vi "Backup get fpga resource ref from channels.vi"(0 "bitfile ref in":refnum<k20>, 5 "channel":refnum<class "TBM channel.lvclass">, 11 "error in (no error)":errorcluster) -> (4 "control ref out":refnum<k20>, 6 "fpga res type":T1, 15 "error out":errorcluster)   [LabVIEW 2015]
uses:
  <vilib>/NI/Tag Bus Module Framework/channel/TBM channel.lvclass
  configuration/fpga resource supported data types.ctl
  fpga channel/fpga channel.lvclass
  <vilib>/NI/Tag Bus/tag/tag descriptor.lvclass/tag descriptor.ctl
  fpga channel/fpga channel.lvclass/fpga channel.ctl
  FXP I_20_5.ctl
  FXP I_24_5.ctl
  FXP I_24_10.ctl
  <vilib>/NI/LVFPGA Adv Session Resources/OpenByNameSubVI.vi
  <vilib>/NI/Tag Bus/tag/read tag name.vi
  fpga channel/Read FXP type.vi
  <vilib>/NI/Tag Bus/tag/read data type.vi
  <vilib>/rvi/interface/common/dynamic/niFpgaEscapeDelimiterAndNull.vi
  <vilib>/Utility/error.llb/Error Cluster From Error Code.vi
  <vilib>/NI/LVFPGA Adv Session Resources/OpenByName.xnode
  <vilib>/NI/LVFPGA Adv Session Resources/LVFPGAAdvSessionResources.lvlib
  configuration/io configuration.lvclass
  io runtime.lvclass
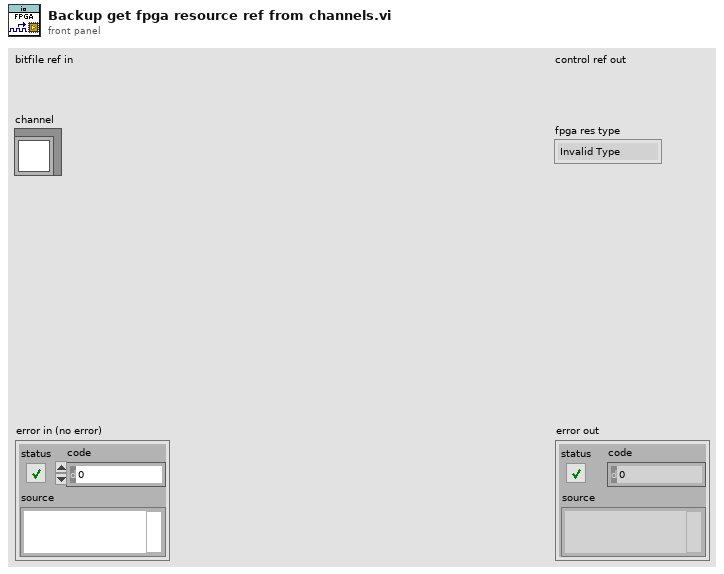
[diagram p1: front panel]
types:
  T1 = typedef "io configuration.lvclass/fpga resource supported data types.ctl" = enum16{"Invalid Type", "Single", "I64", "I32", "I16", "I8", "U64", "U32", "U16", "U8", "Boolean", "FXP I,20,5", "FXP I,24,5", "FXP I,24,10", "Array of I16"}
  T2 = cluster{"Name":string, "Depth":u32, "Write? (Deprecated:Use Implementation)":bool, "Physical Channel":u32, "Base Address":u32, "Data Width":u32, "Data Type":enum32{"Boolean", "I8", "I16", "I32", "I64", "U8", "U16", "U32", "U64", "FXP", "CustomControl", "SGL"}, "FXP Properties":variant, "Write Window Address":u32, "Implementation":enum16{"niFpgaTargetToHost", "niFpgaHostToTarget", "niFpgaPeerToPeerWriter", "niFpgaPeerToPeerReader", "niCoreTargetToHost", "niCoreHostToTarget"}, "Control Set":u32}[]
  T3 = cluster{"Name":string, "type":variant, "indicator?":bool}[]
  T4 = typedef "LVFixedPointRepBitsTypeDef.ctl" = cluster{"Signed":bool, "Word Length":u32, "Integer Word Length":i32}
  T5 = typedef "io runtime.lvclass/FXP I_20_5.ctl" = refnum<k20>
  T6 = typedef "io runtime.lvclass/FXP I_24_5.ctl" = refnum<k20>
  T7 = typedef "io runtime.lvclass/FXP I_24_10.ctl" = refnum<k20>
  T8 = typedef "tag bus.lvlib/tag descriptor.lvclass/Data Type.ctl" = enum16{"Double", "Single", "I64", "I32", "I16", "I8", "U64", "U32", "U16", "U8", "Boolean", "String", "Array of Double", "Array of Single", "Array of I64", "Array of I32", "Array of I16", "Array of I8", "Array of U64", "Array of U32", "Array of U16", "Array of U8", "Array of Boolean", "Array of String"}
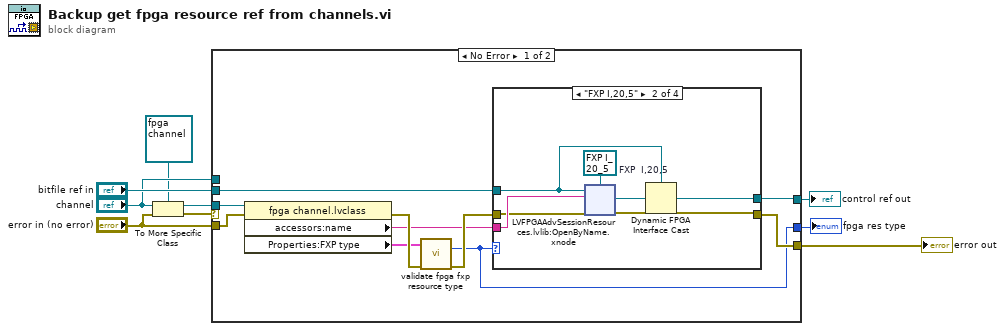
[diagram p0: block diagram]
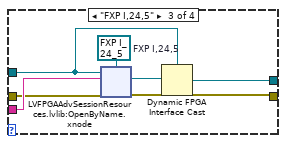
[diagram p3: hidden frame]
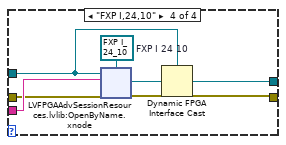
[diagram p4: hidden frame]
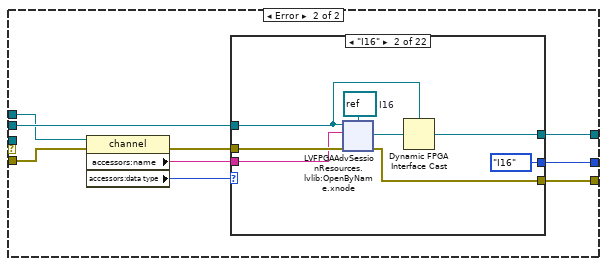
[diagram p5: hidden frame]
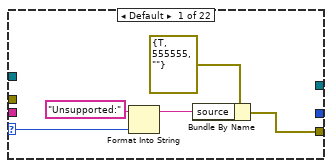
[diagram p6: hidden frame]
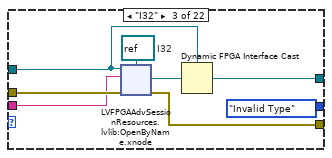
[diagram p7: hidden frame]
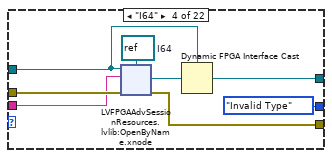
[diagram p8: hidden frame]
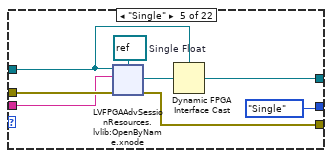
[diagram p9: hidden frame]
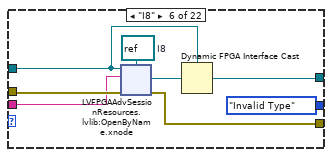
[diagram p10: hidden frame]
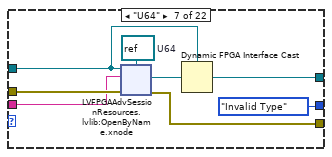
[diagram p11: hidden frame]
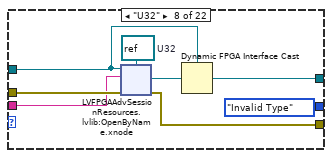
[diagram p12: hidden frame]
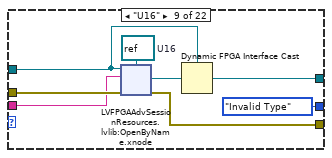
[diagram p13: hidden frame]
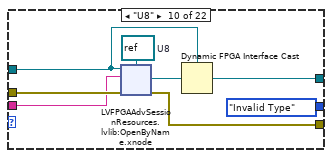
[diagram p14: hidden frame]
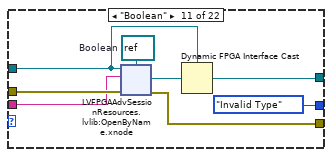
[diagram p15: hidden frame]
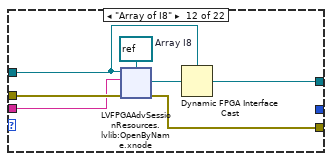
[diagram p16: hidden frame]
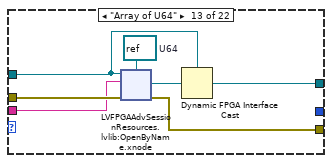
[diagram p17: hidden frame]
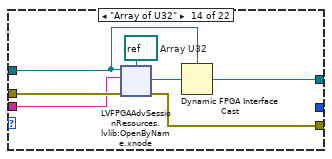
[diagram p18: hidden frame]
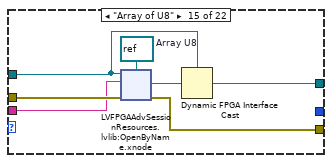
[diagram p19: hidden frame]
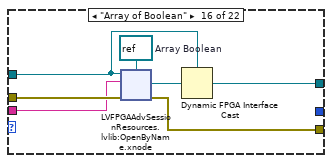
[diagram p20: hidden frame]
diagram:
  n1 = To More Specific Class(target class=refnum<class "fpga channel.lvclass"> refnum ("Fxp Channel.lvclass"), reference="channel", error in="error in (no error)") -> (specific class reference=w8:refnum<class "fpga channel.lvclass">, error out=w9:errorcluster)
  n2 = case shown="No Error" w9 {
    tunnel: w8 -> [w17 _]
    tunnel: "bitfile ref in" -> [w16 w84]
    tunnel: [w13 w85] -> w2
    tunnel: [w15 w89] -> w5
    tunnel: [w11 w81] -> w6
    tunnel: "channel" -> [_ w83]
    tunnel: "error in (no error)" -> [w10 w82]
    frame No Error {
      n3 = property class="fpga channel.lvclass"(reference=w17, error in=w10) -> (error out=w19:errorcluster, "accessors:name"=w14:string, "Properties:FXP type"=w12:T4)  [unwired: 1 out]
      n4 = call "validate fpga fxp resource type.vi"("FXP Representation"=w12, "error in (no error)"=w19) -> ("fpga res type"=w11:T1, "error out"=w18:errorcluster)  [unwired: 11 in, 1 out]
      n5 = case shown="\"FXP I,20,5\"" w11 {
        tunnel: w16 -> [_ w22 w47 w66]
        tunnel: [_ w26 w46 w65] -> w15
        tunnel: w14 -> [_ w25 w45 w64]
        tunnel: w18 -> [w20 w24 w44 w63]
        tunnel: [w20 w23 w43 w62] -> w13
        frame "Invalid Type", Default {
        }
        frame "FXP I,20,5" {
          w21 = T5 refnum  # FXP  I,20,5
          n6 = xnode "LVFPGAAdvSessionResources.lvlib:OpenByName.xnode"("FPGA VI Reference in"=w22, "Resource name in"=w25, "Single resource reference type in"=w21, "Error in"=w24) -> ("Single resource reference out"=w27:T5, "Error out"=w23:errorcluster)  [unwired: 1 out]
          n7 = Dynamic FPGA Interface Cast(Session In=w22, Type=w27) -> (Session Out=w26:refnum<k20>)
        }
        frame "FXP I,24,5" {
          w41 = T6 refnum  # FXP I,24,5
          n8 = xnode "LVFPGAAdvSessionResources.lvlib:OpenByName.xnode"("FPGA VI Reference in"=w47, "Resource name in"=w45, "Single resource reference type in"=w41, "Error in"=w44) -> ("Single resource reference out"=w42:T6, "Error out"=w43:errorcluster)  [unwired: 1 out]
          n9 = Dynamic FPGA Interface Cast(Session In=w47, Type=w42) -> (Session Out=w46:refnum<k20>)
        }
        frame "FXP I,24,10" {
          w61 = T7 refnum  # FXP I 24 10
          n10 = xnode "LVFPGAAdvSessionResources.lvlib:OpenByName.xnode"("FPGA VI Reference in"=w66, "Resource name in"=w64, "Single resource reference type in"=w61, "Error in"=w63) -> ("Single resource reference out"=w67:T7, "Error out"=w62:errorcluster)  [unwired: 1 out]
          n11 = Dynamic FPGA Interface Cast(Session In=w66, Type=w67) -> (Session Out=w65:refnum<k20>)
        }
      }
    }
    frame Error {
      n12 = property class="channel"(reference=w83, error in=w82) -> (error out=w88:errorcluster, "accessors:name"=w86:string, "accessors:data type"=w87:T8)  [unwired: 1 out]
      n13 = case shown="\"I16\"" w87 {
        selector: w87 -> [w92 _ _ _ _ _ _ _ _ _ _ _ _ _ _ _ _ _ _ _ _ _]
        tunnel: w88 -> [_ w102 w123 w144 w165 w186 w207 w228 w249 w270 w291 w311 w331 w351 w371 w391 w411 w431 w451 w471 w491 w511]
        tunnel: [w94 w101 w122 w143 w164 w185 w206 w227 w248 w269 w290 w310 w330 w350 w370 w390 w410 w425 w450 w470 w490 w510] -> w85
        tunnel: w84 -> [_ w99 w120 w141 w162 w183 w204 w225 w246 w267 w288 w308 w328 w348 w368 w388 w407 w428 w447 w467 w487 w507]
        tunnel: w86 -> [_ w100 w121 w142 w163 w184 w205 w226 w247 w268 w289 w309 w329 w349 w369 w389 w409 w430 w449 w469 w489 w509]
        tunnel: [_ w98 w119 w140 w161 w182 w203 w224 w245 w266 w287 w307 w327 w347 w367 w387 w406 w427 w446 w466 w486 w506] -> w89
        tunnel: [_ fpga_resource_supported_data_types."I16" ("fpga res type") fpga_resource_supported_data_types."Invalid Type" ("fpga res type") fpga_resource_supported_data_types."Invalid Type" ("fpga res type") fpga_resource_supported_data_types."Single" ("fpga res type") fpga_resource_supported_data_types."Invalid Type" ("fpga res type") fpga_resource_supported_data_types."Invalid Type" ("fpga res type") fpga_resource_supported_data_types."Invalid Type" ("fpga res type") fpga_resource_supported_data_types."Invalid Type" ("fpga res type") fpga_resource_supported_data_types."Invalid Type" ("fpga res type") fpga_resource_supported_data_types."Invalid Type" ("fpga res type") _ _ _ _ _ _ _ _ _ _ _] -> w81
        frame Default {
          n14 = Format Into String(initial string="Unsupported:" ("source"), w92) -> (resulting string=w90:string)  [unwired: 2 in, 1 out]
          n15 = Bundle By Name(cluster=errorcluster {"status"=TRUE, "code"=555555, "source"=""} ("Error out"), "source"=w90) -> (w94:errorcluster)
        }
        frame "I16" {
          w97 = refnum<k20> refnum  # I16
          n16 = xnode "LVFPGAAdvSessionResources.lvlib:OpenByName.xnode"("FPGA VI Reference in"=w99, "Resource name in"=w100, "Single resource reference type in"=w97, "Error in"=w102) -> ("Single resource reference out"=w96:refnum<k20>, "Error out"=w101:errorcluster)  [unwired: 1 out]
          n17 = Dynamic FPGA Interface Cast(Session In=w99, Type=w96) -> (Session Out=w98:refnum<k20>)
        }
        frame "I32" {
          w118 = refnum<k20> refnum  # I32
          n18 = xnode "LVFPGAAdvSessionResources.lvlib:OpenByName.xnode"("FPGA VI Reference in"=w120, "Resource name in"=w121, "Single resource reference type in"=w118, "Error in"=w123) -> ("Single resource reference out"=w117:refnum<k20>, "Error out"=w122:errorcluster)  [unwired: 1 out]
          n19 = Dynamic FPGA Interface Cast(Session In=w120, Type=w117) -> (Session Out=w119:refnum<k20>)
        }
        frame "I64" {
          w139 = refnum<k20> refnum  # I64
          n20 = xnode "LVFPGAAdvSessionResources.lvlib:OpenByName.xnode"("FPGA VI Reference in"=w141, "Resource name in"=w142, "Single resource reference type in"=w139, "Error in"=w144) -> ("Single resource reference out"=w138:refnum<k20>, "Error out"=w143:errorcluster)  [unwired: 1 out]
          n21 = Dynamic FPGA Interface Cast(Session In=w141, Type=w138) -> (Session Out=w140:refnum<k20>)
        }
        frame "Single" {
          w160 = refnum<k20> refnum  # Single Float
          n22 = xnode "LVFPGAAdvSessionResources.lvlib:OpenByName.xnode"("FPGA VI Reference in"=w162, "Resource name in"=w163, "Single resource reference type in"=w160, "Error in"=w165) -> ("Single resource reference out"=w159:refnum<k20>, "Error out"=w164:errorcluster)  [unwired: 1 out]
          n23 = Dynamic FPGA Interface Cast(Session In=w162, Type=w159) -> (Session Out=w161:refnum<k20>)
        }
        frame "I8" {
          w181 = refnum<k20> refnum  # I8
          n24 = xnode "LVFPGAAdvSessionResources.lvlib:OpenByName.xnode"("FPGA VI Reference in"=w183, "Resource name in"=w184, "Single resource reference type in"=w181, "Error in"=w186) -> ("Single resource reference out"=w180:refnum<k20>, "Error out"=w185:errorcluster)  [unwired: 1 out]
          n25 = Dynamic FPGA Interface Cast(Session In=w183, Type=w180) -> (Session Out=w182:refnum<k20>)
        }
        frame "U64" {
          w202 = refnum<k20> refnum  # U64
          n26 = xnode "LVFPGAAdvSessionResources.lvlib:OpenByName.xnode"("FPGA VI Reference in"=w204, "Resource name in"=w205, "Single resource reference type in"=w202, "Error in"=w207) -> ("Single resource reference out"=w201:refnum<k20>, "Error out"=w206:errorcluster)  [unwired: 1 out]
          n27 = Dynamic FPGA Interface Cast(Session In=w204, Type=w201) -> (Session Out=w203:refnum<k20>)
        }
        frame "U32" {
          w223 = refnum<k20> refnum  # U32
          n28 = xnode "LVFPGAAdvSessionResources.lvlib:OpenByName.xnode"("FPGA VI Reference in"=w225, "Resource name in"=w226, "Single resource reference type in"=w223, "Error in"=w228) -> ("Single resource reference out"=w222:refnum<k20>, "Error out"=w227:errorcluster)  [unwired: 1 out]
          n29 = Dynamic FPGA Interface Cast(Session In=w225, Type=w222) -> (Session Out=w224:refnum<k20>)
        }
        frame "U16" {
          w244 = refnum<k20> refnum  # U16
          n30 = xnode "LVFPGAAdvSessionResources.lvlib:OpenByName.xnode"("FPGA VI Reference in"=w246, "Resource name in"=w247, "Single resource reference type in"=w244, "Error in"=w249) -> ("Single resource reference out"=w243:refnum<k20>, "Error out"=w248:errorcluster)  [unwired: 1 out]
          n31 = Dynamic FPGA Interface Cast(Session In=w246, Type=w243) -> (Session Out=w245:refnum<k20>)
        }
        frame "U8" {
          w265 = refnum<k20> refnum  # U8
          n32 = xnode "LVFPGAAdvSessionResources.lvlib:OpenByName.xnode"("FPGA VI Reference in"=w267, "Resource name in"=w268, "Single resource reference type in"=w265, "Error in"=w270) -> ("Single resource reference out"=w264:refnum<k20>, "Error out"=w269:errorcluster)  [unwired: 1 out]
          n33 = Dynamic FPGA Interface Cast(Session In=w267, Type=w264) -> (Session Out=w266:refnum<k20>)
        }
        frame "Boolean" {
          w286 = refnum<k20> refnum  # Boolean
          n34 = xnode "LVFPGAAdvSessionResources.lvlib:OpenByName.xnode"("FPGA VI Reference in"=w288, "Resource name in"=w289, "Single resource reference type in"=w286, "Error in"=w291) -> ("Single resource reference out"=w285:refnum<k20>, "Error out"=w290:errorcluster)  [unwired: 1 out]
          n35 = Dynamic FPGA Interface Cast(Session In=w288, Type=w285) -> (Session Out=w287:refnum<k20>)
        }
        frame "Array of I8" {
          w305 = refnum<k20> refnum  # Array I8
          n36 = xnode "LVFPGAAdvSessionResources.lvlib:OpenByName.xnode"("FPGA VI Reference in"=w308, "Resource name in"=w309, "Single resource reference type in"=w305, "Error in"=w311) -> ("Single resource reference out"=w306:refnum<k20>, "Error out"=w310:errorcluster)  [unwired: 1 out]
          n37 = Dynamic FPGA Interface Cast(Session In=w308, Type=w306) -> (Session Out=w307:refnum<k20>)
        }
        frame "Array of U64" {
          w325 = refnum<k20> refnum  # U64
          n38 = xnode "LVFPGAAdvSessionResources.lvlib:OpenByName.xnode"("FPGA VI Reference in"=w328, "Resource name in"=w329, "Single resource reference type in"=w325, "Error in"=w331) -> ("Single resource reference out"=w326:refnum<k20>, "Error out"=w330:errorcluster)  [unwired: 1 out]
          n39 = Dynamic FPGA Interface Cast(Session In=w328, Type=w326) -> (Session Out=w327:refnum<k20>)
        }
        frame "Array of U32" {
          w345 = refnum<k20> refnum  # Array U32
          n40 = xnode "LVFPGAAdvSessionResources.lvlib:OpenByName.xnode"("FPGA VI Reference in"=w348, "Resource name in"=w349, "Single resource reference type in"=w345, "Error in"=w351) -> ("Single resource reference out"=w346:refnum<k20>, "Error out"=w350:errorcluster)  [unwired: 1 out]
          n41 = Dynamic FPGA Interface Cast(Session In=w348, Type=w346) -> (Session Out=w347:refnum<k20>)
        }
        frame "Array of U8" {
          w365 = refnum<k20> refnum  # Array U8
          n42 = xnode "LVFPGAAdvSessionResources.lvlib:OpenByName.xnode"("FPGA VI Reference in"=w368, "Resource name in"=w369, "Single resource reference type in"=w365, "Error in"=w371) -> ("Single resource reference out"=w366:refnum<k20>, "Error out"=w370:errorcluster)  [unwired: 1 out]
          n43 = Dynamic FPGA Interface Cast(Session In=w368, Type=w366) -> (Session Out=w367:refnum<k20>)
        }
        frame "Array of Boolean" {
          w385 = refnum<k20> refnum  # Array Boolean
          n44 = xnode "LVFPGAAdvSessionResources.lvlib:OpenByName.xnode"("FPGA VI Reference in"=w388, "Resource name in"=w389, "Single resource reference type in"=w385, "Error in"=w391) -> ("Single resource reference out"=w386:refnum<k20>, "Error out"=w390:errorcluster)  [unwired: 1 out]
          n45 = Dynamic FPGA Interface Cast(Session In=w388, Type=w386) -> (Session Out=w387:refnum<k20>)
        }
        frame "Array of Single" {
          w405 = refnum<k20> refnum  # Array Single
          n46 = xnode "LVFPGAAdvSessionResources.lvlib:OpenByName.xnode"("FPGA VI Reference in"=w407, "Resource name in"=w409, "Single resource reference type in"=w405, "Error in"=w411) -> ("Single resource reference out"=w408:refnum<k20>, "Error out"=w410:errorcluster)  [unwired: 1 out]
          n47 = Dynamic FPGA Interface Cast(Session In=w407, Type=w408) -> (Session Out=w406:refnum<k20>)
        }
        frame "Array of Double" {
          w426 = refnum<k20> refnum  # FXP
          n48 = xnode "LVFPGAAdvSessionResources.lvlib:OpenByName.xnode"("FPGA VI Reference in"=w428, "Resource name in"=w430, "Single resource reference type in"=w426, "Error in"=w431) -> ("Single resource reference out"=w429:refnum<k20>, "Error out"=w425:errorcluster)  [unwired: 1 out]
          n49 = Dynamic FPGA Interface Cast(Session In=w428, Type=w429) -> (Session Out=w427:refnum<k20>)
        }
        frame "Array of I64" {
          w445 = refnum<k20> refnum  # Array I64
          n50 = xnode "LVFPGAAdvSessionResources.lvlib:OpenByName.xnode"("FPGA VI Reference in"=w447, "Resource name in"=w449, "Single resource reference type in"=w445, "Error in"=w451) -> ("Single resource reference out"=w448:refnum<k20>, "Error out"=w450:errorcluster)  [unwired: 1 out]
          n51 = Dynamic FPGA Interface Cast(Session In=w447, Type=w448) -> (Session Out=w446:refnum<k20>)
        }
        frame "Array of I32" {
          w465 = refnum<k20> refnum  # Array I32
          n52 = xnode "LVFPGAAdvSessionResources.lvlib:OpenByName.xnode"("FPGA VI Reference in"=w467, "Resource name in"=w469, "Single resource reference type in"=w465, "Error in"=w471) -> ("Single resource reference out"=w468:refnum<k20>, "Error out"=w470:errorcluster)  [unwired: 1 out]
          n53 = Dynamic FPGA Interface Cast(Session In=w467, Type=w468) -> (Session Out=w466:refnum<k20>)
        }
        frame "Array of I16" {
          w485 = refnum<k20> refnum  # Array I16
          n54 = xnode "LVFPGAAdvSessionResources.lvlib:OpenByName.xnode"("FPGA VI Reference in"=w487, "Resource name in"=w489, "Single resource reference type in"=w485, "Error in"=w491) -> ("Single resource reference out"=w488:refnum<k20>, "Error out"=w490:errorcluster)  [unwired: 1 out]
          n55 = Dynamic FPGA Interface Cast(Session In=w487, Type=w488) -> (Session Out=w486:refnum<k20>)
        }
        frame "Array of U16" {
          w505 = refnum<k20> refnum  # Array U16
          n56 = xnode "LVFPGAAdvSessionResources.lvlib:OpenByName.xnode"("FPGA VI Reference in"=w507, "Resource name in"=w509, "Single resource reference type in"=w505, "Error in"=w511) -> ("Single resource reference out"=w508:refnum<k20>, "Error out"=w510:errorcluster)  [unwired: 1 out]
          n57 = Dynamic FPGA Interface Cast(Session In=w507, Type=w508) -> (Session Out=w506:refnum<k20>)
        }
      }
    }
  }
  "error out" <- w2
  "control ref out" <- w5
  "fpga res type" <- w6
